vi "CheckError.vi"(8 "error in (no error)":errorcluster, 10 "timeout?":bool, 11 "dynamic fgpa vi reference in":T1) -> (0 "error out":errorcluster, 3 "dynamic fpga vi reference out":T1)   [LabVIEW 2017, in "cRIOWfmLibMcsa.lvlib"]
uses:
  <vilib>/addons/InsightCM/Devices/Shared/Mcsa/cRIOWfmAcqMcsa/cRIOWfmLibMcsa.lvlib
  <vilib>/addons/InsightCM/Devices/Shared/Mcsa/cRIOWfmAcqMcsa/controls/rwfm_DynamicFPGArefMCSA.ctl
  <vilib>/Utility/error.llb/Error Cluster From Error Code.vi
  <vilib>/rvi/errors/niLvFpgaAdjustHostInterfaceError.vi
  <vilib>/rvi/interface/nirviReadWriteControl/nirviReadWriteControl.xnode
  <vilib>/addons/InsightCM/Devices/Shared/Cms/cRIOWfmAcq/cRIOWfmLib.lvlib
  <vilib>/rvi/interface/Simulation/niFpgaSimulationCallBeginRW.vi
  NiFpgaLv.dll
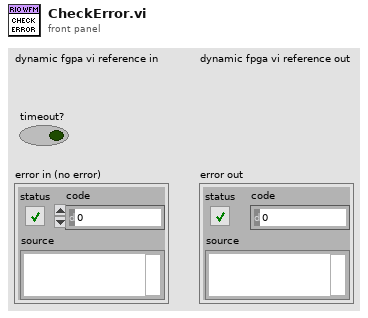
[diagram p1: front panel]
types:
  T1 = typedef "cRIOWfmLibMcsa.lvlib/rwfm_DynamicFPGArefMCSA.ctl" = refnum<k20>
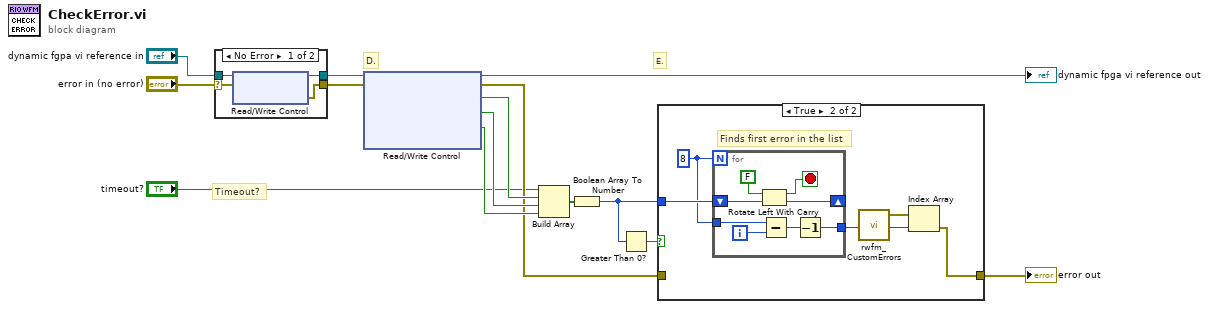
[diagram p0: block diagram]
diagram:
  # "E."
  # "D."
  # "Timeout?"
  n1 = case shown="No Error" "error in (no error)" {
    selector: "error in (no error)" -> [w16 w20]
    tunnel: "dynamic fgpa vi reference in" -> [w18 w19]
    tunnel: [w17 w19] -> w7
    tunnel: [w15 w20] -> w8
    frame No Error {
      n2 = xnode "Read/Write Control"("FPGA VI Reference In"=w18, "error in"=w16) -> ("FPGA VI Reference Out"=w17:T1, "FPGA Error"=w15:errorcluster)  [unwired: 1 out]
    }
    frame Error {
    }
  }
  n3 = xnode "Read/Write Control"("FPGA VI Reference In"=w7, "error in"=w8) -> ("FPGA VI Reference Out"=→"dynamic fpga vi reference out":T1, "error out"=w5:errorcluster, "Module Underflow"=w12:bool, "DMA FIFO Full"=w13:bool, "Chan Count"=w14:bool)  [unwired: 1 out]
  n4 = Build Array("timeout?", w12, w13, w14) -> (w3:bool[])
  n5 = Boolean Array To Number(Boolean array=w3) -> (number=w1:u8)
  n6 = Greater Than 0?(x=w1) -> (x > 0?=w2:bool)
  n7 = case shown="True" w2 {
    tunnel: w1 -> [_ w26]
    tunnel: [w21 w22] -> w11
    tunnel: w5 -> [w21 _]
    frame False {
    }
    frame True {
      w24 = 8
      # "Finds first error in the list"
      n8 = for {
        N: w24 -> [_]
        tunnel: [w28] -> w25
        tunnel: w24 -> [w31]
        shift-right: [w27] -> _
        shift-left: w26 -> [w34]
        i -> [w30]
        stop <- w33 stop-if-true
        n9 = Rotate Left With Carry(2:w34, 3:FALSE ("carry")) -> (0:w27:u8, 1:w33:bool)
        n10 = Subtract(x=w31, y=w30) -> (x-y=w29:i32)
        n11 = Decrement(x=w29) -> (x-1=w28:i32)
      }
      n12 = call <vilib>:"rwfm_CustomErrors.vi"() -> ("Error Array"=w23:errorcluster[])  [unwired: 5 in]
      n13 = Index Array(array=w23, index=w25) -> (element=w22:errorcluster)
    }
  }
  "error out" <- w11
